vi "Close.vi"(8 "error in (no error)":errorcluster, 11 "KUKA youBot wheel motor in":refnum<class "NI_Robotics_KUKA youBot Wheel Motor.lvclass">) -> (0 "error out":errorcluster)   [LabVIEW 2017, in "NI_Robotics_KUKA youBot Host.lvlib" / "NI_Robotics_KUKA youBot Wheel Motor.lvclass"]
uses:
  <vilib>/robotics/KUKA youBot/Motor/Wheel Motor/NI_Robotics_KUKA youBot Wheel Motor.lvclass
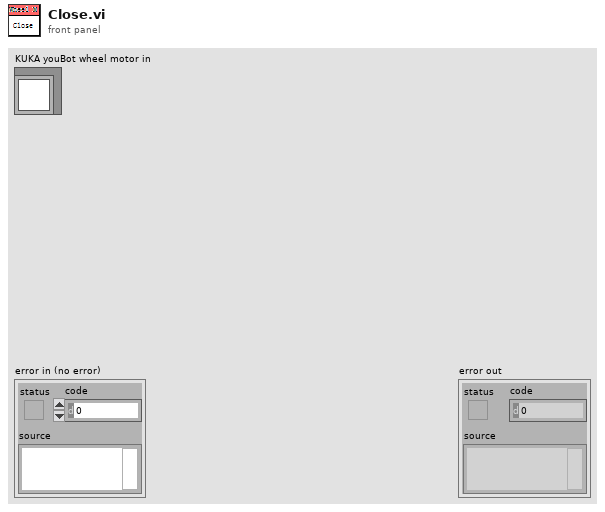
[diagram p1: front panel]
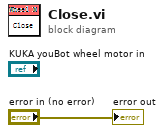
[diagram p0: block diagram]
diagram:
  "error out" <- "error in (no error)"
